vi "Handle Event.vi"(8 "error in (no error)":errorcluster, 10 "Event":T1={"Level"=enum."Info", "Context"="", "Message"="", "Error"={"status"=FALSE, "code"=0, "source"=""}, "Time Stamp"=timestamp(0 s since 1904-01-01)}, 11 "BasicEventLogger in":refnum<class "BasicEventLogger.lvclass">) -> (0 "error out":errorcluster, 3 "BasicEventLogger out":refnum<class "BasicEventLogger.lvclass">)   [LabVIEW 2020, in "Volatus.lvlib" / "BasicEventLogger.lvclass"]
uses:
  BasicEventLogger.lvclass
  Event.ctl
  Event Level.ctl
  BasicEventLogger.lvclass/BasicEventLogger.ctl
  Volatus.lvlib
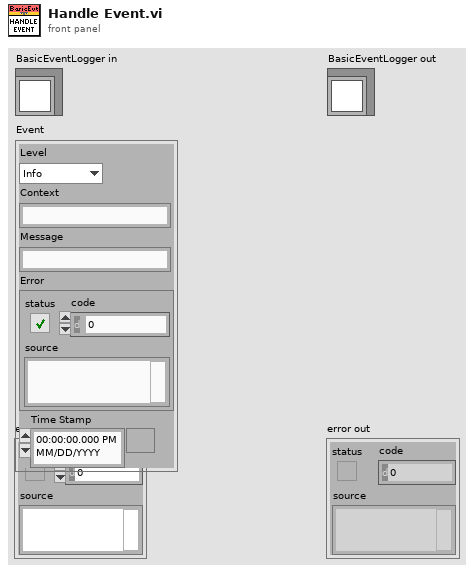
[diagram p1: front panel]
types:
  T1 = typedef "Volatus.lvlib/Event.ctl" = cluster{"Level":T2, "Context":string, "Message":string, "Error":errorcluster, "Time Stamp":timestamp}
  T2 = typedef "Volatus.lvlib/Event Level.ctl" = enum16{"Debug", "Info", "Warning", "Error"}
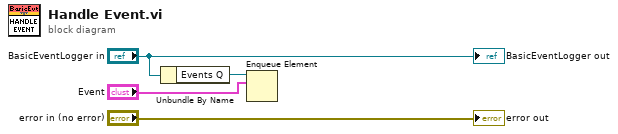
[diagram p0: block diagram]
diagram:
  n1 = Unbundle By Name("BasicEventLogger in") -> ("Events Q"=w2:refnum<queue>)
  n2 = Enqueue Element(queue=w2, element="Event") -> ()  [unwired: 2 in, 3 out]
  "error out" <- "error in (no error)"
  "BasicEventLogger out" <- "BasicEventLogger in"
